vi "Agilent VNA Set Trace.vi"(7 "Agilent VNA":T1, 8 "error in (no error)":errorcluster, 9 "Trace":i8=1 min=1 max=99 step=1, 10 "Channel":i8=1 min=1 max=99 step=1, 11 "VISA Resource Name":refnum<visa-resource-name>) -> (0 "error out":errorcluster, 3 "dup VISA Resource Name":refnum<visa-resource-name>)   [LabVIEW 2011]
uses:
  TypeDefs/Agilent VNA Instrument Info.ctl
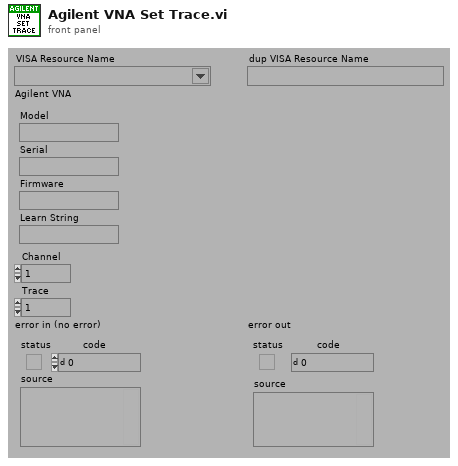
[diagram p1: front panel]
types:
  T1 = typedef "Agilent VNA Instrument Info.ctl" = cluster{"Model":string, "Serial":string, "Firmware":string, "Learn String":string}
  T2 = typedef "Agilent VNA Model.ctl" = enum16{"Not Supported", "8510X", "8719X", "8720X", "8722X", "8753X", "ENA", "PNA", "Field Fox"}
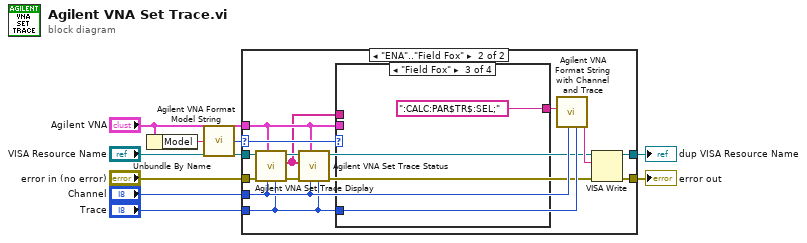
[diagram p0: block diagram]
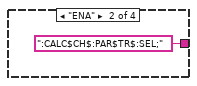
[diagram p4: hidden frame]
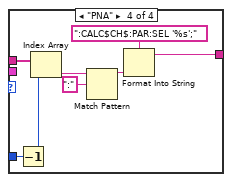
[diagram p5: hidden frame]
diagram:
  n1 = Unbundle By Name("Agilent VNA") -> ("Model"=w3:string)
  n2 = call "Agilent VNA Format Model String.vi"("Model"=w3) -> ("Model"=w1:T2)
  n3 = case shown="\"ENA\"..\"Field Fox\"" w1 {
    selector: w1 -> [_ w22]
    tunnel: [w11 w26] -> w9
    tunnel: [w10 w25] -> w8
    tunnel: "VISA Resource Name" -> [w11 w21]
    tunnel: "error in (no error)" -> [w10 w20]
    tunnel: "Trace" -> [_ w15]
    tunnel: "Channel" -> [_ w16]
    tunnel: "Agilent VNA" -> [_ w17]
    frame "Not Supported".."8753X" {
    }
    frame "ENA".."Field Fox" {
      n4 = call "Agilent VNA Set Trace Display.vi"("Trace"=w15, "Channel"=w16, "Agilent VNA"=w17, "error in (no error)"=w20, "VISA Resource Name"=w21) -> ("error out"=w18:errorcluster, "Measurements"=w12:string[], "dup VISA Resource Name"=w19:refnum<visa-resource-name>)  [unwired: 4 out]
      n5 = call "Agilent VNA Set Trace Status.vi"("Trace"=w15, "Channel"=w16, "Agilent VNA"=w17, "error in (no error)"=w18, "Measurements"=w12, "VISA Resource Name"=w19) -> ("error out"=w13:errorcluster, "dup VISA Resource Name"=w14:refnum<visa-resource-name>)  [unwired: 4 out]
      n6 = case shown="\"Field Fox\"" w22 {
        tunnel: [_ ":CALC$CH$:PAR$TR$:SEL;" ":CALC:PAR$TR$:SEL;" w33] -> w23
        tunnel: w17 -> [_ _ _ _]
        tunnel: w15 -> [_ _ _ w36]
        tunnel: w12 -> [_ _ _ w32]
        frame "Not Supported".."8753X" {
        }
        frame "ENA" {
        }
        frame "Field Fox" {
        }
        frame "PNA" {
          n7 = Decrement(x=w36) -> (x-1=w35:i8)
          n8 = Index Array(array=w32, index=w35) -> (element=w31:string)
          n9 = Match Pattern(string=w31, regular expression=":") -> (before substring=w30:string)  [unwired: 1 in, 3 out]
          n10 = Format Into String(format string=":CALC$CH$:PAR:SEL '%s';", w30) -> (resulting string=w33:string)  [unwired: 2 in, 1 out]
        }
      }
      n11 = call "Agilent VNA Format String with Channel and Trace.vi"("Trace"=w15, "Channel"=w16, "String"=w23) -> ("String Out"=w24:string)  [unwired: 6 out]
      n12 = VISA Write(VISA resource name=w14, write buffer=w24, error in (no error)=w13) -> (VISA resource name out=w26:refnum<visa-resource-name>, error out=w25:errorcluster)  [unwired: 1 out]
    }
  }
  "dup VISA Resource Name" <- w9
  "error out" <- w8
